vi "Set New Selection to End.vi"(8 "error in (no error)":errorcluster, 11 ".NET Refnum in":refnum<k24>) -> (0 "error out":errorcluster, 1 "Current SelectionLength":i32, 2 "Current SelectionStart":i32, 3 ".NET Refnum out":refnum<k24>, 4 "Current Selection at End?":bool, 6 "New SelectionStart: End of RTB":i32)   [LabVIEW 2019, in "Rich Text Box.lvlib"]
uses:
  Rich Text Box.lvlib
  System.Windows.Forms
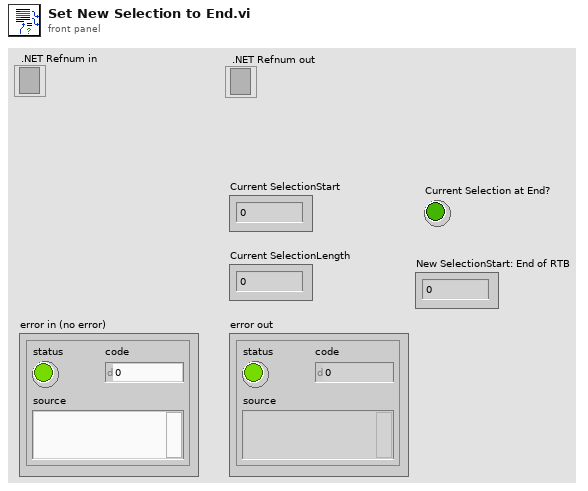
[diagram p1: front panel]
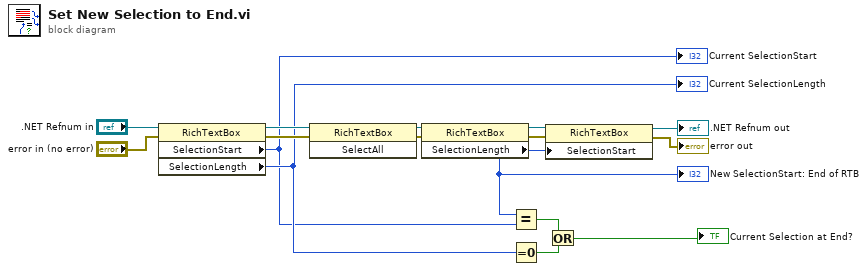
[diagram p0: block diagram]
diagram:
  n1 = property class="RichTextBox"(reference=".NET Refnum in", error in="error in (no error)") -> (reference out=w15:refnum<k24>, error out=w16:errorcluster, "SelectionStart"=w5:i32, "SelectionLength"=w6:i32)
  "Current SelectionLength" <- w6
  "Current SelectionStart" <- w5
  n2 = invoke class="RichTextBox" method="SelectAll"(reference=w15, error in=w16) -> (reference out=w9:refnum<k24>, error out=w10:errorcluster)  [unwired: 1 in, 1 out]
  n3 = property class="RichTextBox"(reference=w9, error in=w10) -> (reference out=w11:refnum<k24>, error out=w12:errorcluster, "SelectionLength"=w4:i32)
  "New SelectionStart: End of RTB" <- w4
  n4 = Equal?(x=w4, y=w5) -> (x = y?=w3:bool)
  n5 = Equal To 0?(x=w6) -> (x = 0?=w2:bool)
  n6 = property class="RichTextBox"(reference=w11, error in=w12, "SelectionStart"=w4) -> (reference out=→".NET Refnum out":refnum<k24>, error out=→"error out":errorcluster)
  n7 = Or(x=w3, y=w2) -> (x .or. y?=→"Current Selection at End?":bool)
